vi "QMH Add Message to Queue (Single Element).vi"(6 "Insert (T)":bool=TRUE, 7 "At Front (F)":bool, 8 "error in (no error)":errorcluster, 9 "Parameter":string, 10 "Message":string, 11 "queue in":refnum<queue>) -> (0 "error out":errorcluster, 3 "queue out":refnum<queue>)   [LabVIEW 2013, in "QHM.lvlib"]
doc: "Place elements wired to the \"elements\" input on the event queue."
uses:
  QHM.lvlib
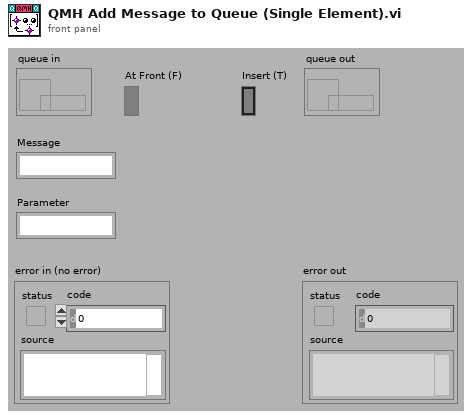
[diagram p1: front panel]
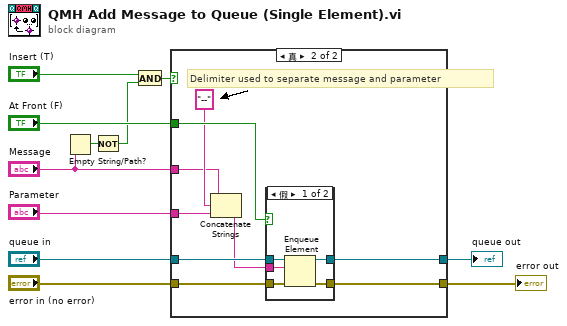
[diagram p0: block diagram]
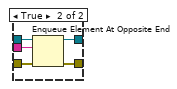
[diagram p3: hidden frame]
diagram:
  n1 = Empty String/Path?(string/path="Message") -> (empty?=w2:bool)
  n2 = Not(x=w2) -> (.not. x?=w1:bool)
  n3 = And(x="Insert (T)", y=w1) -> (x .and. y?=w5:bool)
  n4 = case shown="真" w5 {
    tunnel: "error in (no error)" -> [w12 w22]
    tunnel: [w12 w21] -> w10
    tunnel: "queue in" -> [w13 w20]
    tunnel: [w13 w19] -> w8
    tunnel: "At Front (F)" -> [_ w18]
    tunnel: "Message" -> [_ w15]
    tunnel: "Parameter" -> [_ w14]
    frame False {
    }
    frame True {
      # "Delimiter used to separate message and parameter"
      n5 = Concatenate Strings(w15, "--" ("string"), w14) -> (w16:string)
      n6 = case shown="假" w18 {
        tunnel: w16 -> [w27 w32]
        tunnel: w20 -> [w26 w28]
        tunnel: [w25 w29] -> w19
        tunnel: [w24 w30] -> w21
        tunnel: w22 -> [w23 w31]
        frame False {
          n7 = Enqueue Element(queue=w26, element=w27, error in (no error)=w23) -> (queue out=w25:refnum<queue>, error out=w24:errorcluster)  [unwired: 1 in, 1 out]
        }
        frame True {
          n8 = Enqueue Element At Opposite End(queue=w28, element=w32, error in (no error)=w31) -> (queue out=w29:refnum<queue>, error out=w30:errorcluster)  [unwired: 1 in, 1 out]
        }
      }
    }
  }
  "error out" <- w10
  "queue out" <- w8
